vi "Receive Message.vi"(6 "priority":i32, 10 "Data Repository in":refnum<class "Data Repository.lvclass">, 11 "Message in":refnum<class "Message.lvclass">) -> (0 "error out":errorcluster, 2 "Actor out":refnum<class "Actor.lvclass">)   [LabVIEW 2020, in "Data Repository.lvlib" / "Data Repository.lvclass"]
doc: "Filters for Data messages and send/store these on named notifiers (named by Data alias). All other messages are handled normally.\n\nData is only sent/stored when the exception state is valid and the Data alias is non empty."
uses:
  Data Repository.lvclass
  PPL/HDH.Actor Framework.Core.Actor.lvlibp/1abvi3w/vi.lib/ActorFramework/Message/Message.lvclass
  PPL/HDH.Actor Framework.Core.Actor.lvlibp/1abvi3w/vi.lib/ActorFramework/Actor/Actor.lvclass
  C:/Current projects/WS/PPL/HDH.Actor Framework.Core.Actor.lvlibp/1abvi3w/vi.lib/ActorFramework/Actor/Actor.lvclass
  PPL/HDH.Actor Framework.Core.Publisher.lvlibp/Messages/Data Msg/Data Msg.lvclass
  Data Repository.lvclass/Data Repository.ctl
  PPL/HDH.Data.Generic.lvlibp/Synchronization/Notifier/Notifier.lvclass
  PPL/HDH.Data.Generic.lvlibp/Data.lvclass
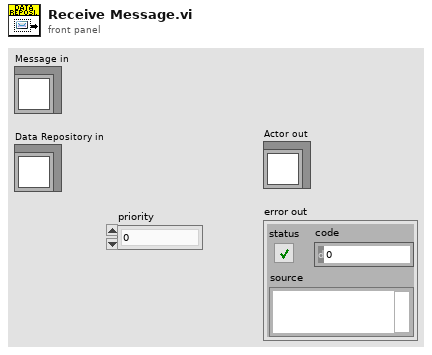
[diagram p1: front panel]
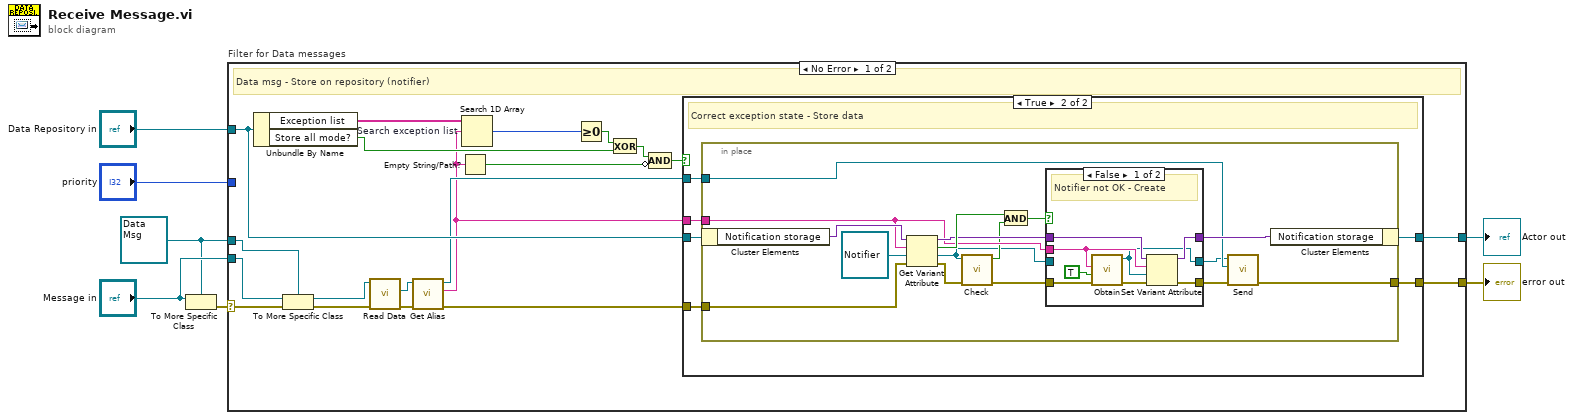
[diagram p0: block diagram]
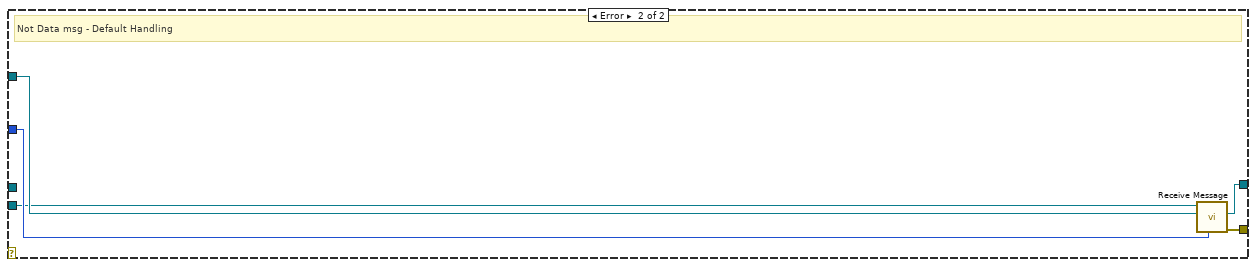
[diagram p4: hidden frame]
diagram:
  w1 = refnum<class "Data Msg.lvclass"> refnum ("HDH.Actor Framework.Core.Publisher.lvlibp:Data Msg.lvclass")
  n1 = To More Specific Class(target class=w1, reference="Message in") -> (error out=w3:errorcluster)  [unwired: 1 in, 1 out]
  n2 = case "Filter for Data messages" shown="No Error" w3 {
    selector: w3 -> [w25 _]
    tunnel: [w12 w67] -> w7
    tunnel: [w15 w66] -> w6
    tunnel: "priority" -> [_ w65]
    tunnel: "Data Repository in" -> [w16 w64]
    tunnel: "Message in" -> [w27 w63]
    tunnel: w1 -> [w26 _]
    frame No Error {
      # "Data msg - Store on repository (notifier)"
      n3 = Unbundle By Name(w16) -> ("Exception list"=w21:string[], "Store all mode?"=w17:bool)
      n4 = To More Specific Class(target class=w26, reference=w27, error in=w25) -> (specific class reference=w24:refnum<class "Data Msg.lvclass">, error out=w23:errorcluster)
      n5 = call "Read Data.vi"("error in (no error)"=w23, "Data Msg in"=w24) -> ("error out"=w20:errorcluster, "Data"=w22:refnum<class "Data.lvclass">)  [unwired: 7 in, 1 out]
      n6 = call-dynamic "Get Alias.vi"("error in (no error)"=w20, "Data in"=w22) -> ("error out"=w13:errorcluster, "Alias"=w11:string, "Data out"=w14:refnum<class "Data.lvclass">)  [unwired: 7 in]
      n7 = Empty String/Path?(string/path=w11) -> (empty?=w9:bool)
      n8 = Search 1D Array "Search exception list"(1D array=w21, element=w11) -> (index of element=w19:i32)  [unwired: 1 in]
      n9 = Greater Or Equal To 0?(x=w19) -> (x >= 0?=w18:bool)
      n10 = Exclusive Or(1:w17, 2:w18) -> (0:w10:bool)
      n11 = Compound Arithmetic op=AND(w10, invert w9) -> (w8:bool)
      n12 = case shown="True" w8 {
        tunnel: w16 -> [w29 w35]
        tunnel: [w29 w34] -> w15
        tunnel: w14 -> [_ w31]
        tunnel: w13 -> [w28 w32]
        tunnel: [w28 w30] -> w12
        tunnel: w11 -> [_ w33]
        frame False {
          # "Incorrect exception state - Don't store data"
        }
        frame True {
          # "Correct exception state - Store data"
          n13 = in-place {
            in-place-border: w33 -> [w46]
            in-place-border: w32 -> [w47]
            in-place-border: w31 -> [w39]
            in-place-border: [w36] -> w30
            n14 = in-place-cluster #1(w35) -> ("Notification storage"=w51:variant)
            n15 = Get Variant Attribute(Variant=w51, name=w46, default value (empty Variant)=refnum<class "Notifier.lvclass"> refnum ("HDH.Data.Generic.lvlibp:Notifier.lvclass"), error in=w47) -> (duplicate Variant=w48:variant, found=w49:bool, value=w41:refnum<class "Notifier.lvclass">, error out=w45:errorcluster)
            n16 = call "Check.vi"("error in (no error)"=w45, "Notifier in"=w41) -> ("error out"=w44:errorcluster, "Notifier is valid?"=w42:bool)  [unwired: 8 in]
            n17 = And(x=w49, y=w42) -> (x .and. y?=w43:bool)
            n18 = case shown="False" w43 {
              tunnel: w48 -> [w56 w62]
              tunnel: [w55 w62] -> w40
              tunnel: [w52 w61] -> w38
              tunnel: w44 -> [w58 w61]
              tunnel: w46 -> [w57 _]
              tunnel: [w53 w60] -> w37
              tunnel: w41 -> [_ w60]
              frame False {
                # "Notifier not OK - Create"
                n19 = call "Obtain.vi"("error in (no error)"=w58, "create if not found? (T)"=TRUE, "Name (\"\")"=w57) -> ("error out"=w54:errorcluster, "Notifier out"=w53:refnum<class "Notifier.lvclass">)  [unwired: 6 in, 1 out]
                n20 = Set Variant Attribute(Variant=w56, name=w57, value=w53, error in=w54) -> (Variant out=w55:variant, error out=w52:errorcluster)  [unwired: 1 out]
              }
              frame True {
                # "Notifier OK - Skip"
              }
            }
            n21 = call "Send.vi"("error in (no error)"=w38, "Data Notification"=w39, "Notifier in"=w37) -> ("error out"=w36:errorcluster)  [unwired: 7 in, 1 out]
            n22 = in-place-cluster #1("Notification storage"=w40) -> (w34:refnum<class "Data Repository.lvclass">)
          }
        }
      }
    }
    frame Error {
      # "Not Data msg - Default Handling"
      n23 = call-parent "Receive Message.vi"("priority"=w65, "Actor in"=w64, "Message in"=w63) -> ("error out"=w67:errorcluster, "Actor out"=w66:refnum<class "Actor.lvclass">)  [unwired: 7 in]
    }
  }
  "error out" <- w7
  "Actor out" <- w6
